vi "SEA_9811_ARINCdata2word.vi"(7 "Reverse label bits":bool, 8 "error in (no error)":errorcluster, 11 "ARINC word in":T1 {"ARINC word" format="%032b"}) -> (0 "error out":errorcluster, 3 "ARINC word out":T2 format="%032b")   [LabVIEW 2012]
uses:
  Typdefs/ARINC word.ctl
  Typdefs/ARINC word cluster.ctl
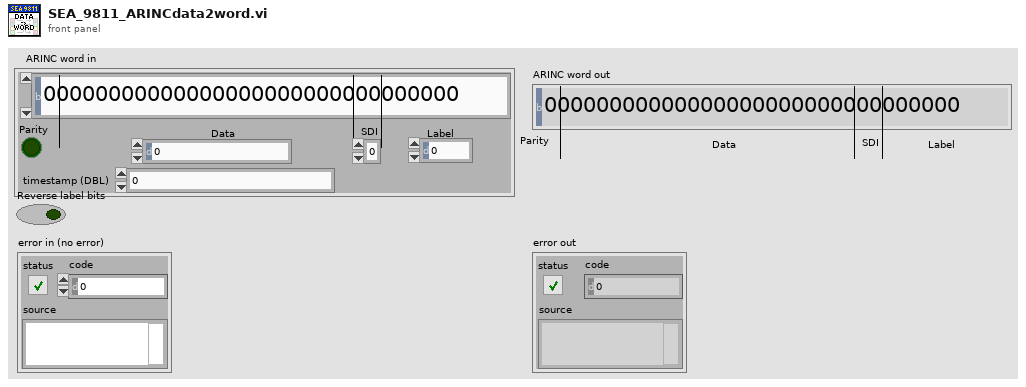
[diagram p1: front panel]
types:
  T1 = typedef "ARINC word cluster.ctl" = cluster{"ARINC word":T2, "Label":u8, "SDI":u8, "Data":u32, "Parity":bool, "timestamp (DBL)":dbl}
  T2 = typedef "ARINC word.ctl" = u32
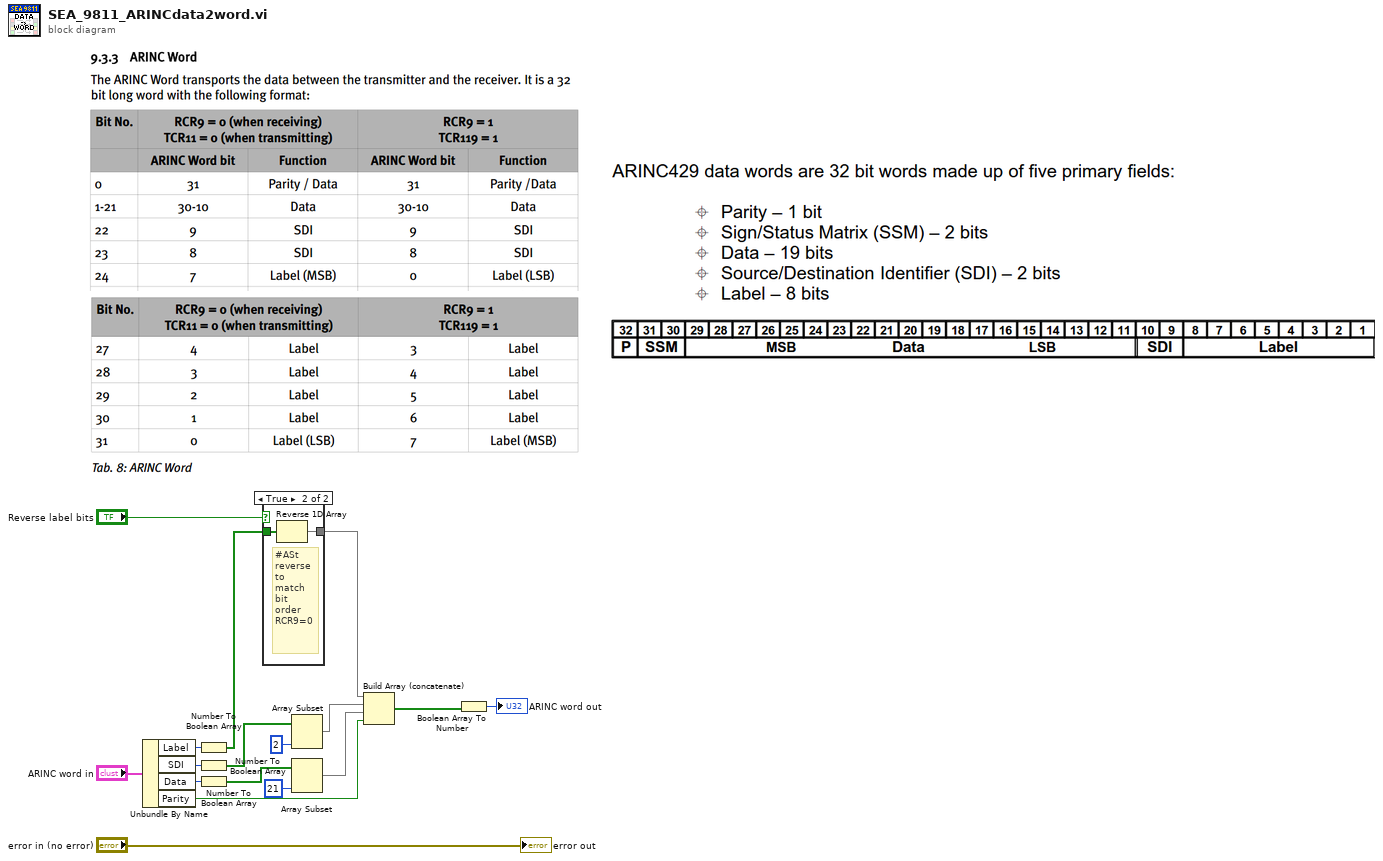
[diagram p0: block diagram]
diagram:
  n1 = Unbundle By Name("ARINC word in") -> ("Label"=w14:u8, "SDI"=w2:u8, "Data"=w3:u32, "Parity"=w5:bool)
  n2 = Number To Boolean Array(number=w14) -> (Boolean array=w13:bool[])
  n3 = Number To Boolean Array(number=w2) -> (Boolean array=w9:bool[])
  n4 = Number To Boolean Array(number=w3) -> (Boolean array=w12:bool[])
  n5 = case shown="True" "Reverse label bits" {
    tunnel: [w18 w20] -> w6
    tunnel: w13 -> [w18 w19]
    frame False {
    }
    frame True {
      # "#ASt\nreverse\nto \nmatch\nbit\norder\nRCR9=0"
      n6 = Reverse 1D Array(array=w19) -> (reversed array=w20:bool[])
    }
  }
  n7 = Array Subset(array=w9, length=2) -> (w8:bool[])  [unwired: 1 in]
  n8 = Array Subset(array=w12, length=21) -> (w7:bool[])  [unwired: 1 in]
  n9 = Build Array (concatenate)(w6, w8, w7, w5) -> (w4:bool[])
  n10 = Boolean Array To Number(Boolean array=w4) -> (number=→"ARINC word out":u32)
  "error out" <- "error in (no error)"
